vi "Initialize Instrument Engine.vi"(8 "error in (no error)":errorcluster, 9 "Name":string, 11 "Process":refnum<class "Process.lvclass">) -> (0 "error out":errorcluster, 2 "notification":bool, 3 "State Variables":T1)   [LabVIEW 2015, in "Instrument Addon Engine.lvlib"]
uses:
  Instrument Addon Engine.lvlib
  Types/Engine State Variables.ctl
  <vilib>/NI/NIVS Inline Async API/_VS Inline Async API/Process/Process.lvclass
  <vilib>/NI/NIVS Addon Network Comm/Engine/VeriStand Comm.lvclass
  <vilib>/NI/NIVS Inline Async API/_Data Access Engine/Access Type Classes/Write/Write.lvclass
  <vilib>/NI/NIVS Inline Async API/_Data Access Engine/Access Type Classes/Read/Read.lvclass
  <vilib>/NI/NIVS Inline Async API/_Data Access Engine/Access Type Classes/ReadWrite/ReadWrite.lvclass
  <vilib>/NI/NIVS Addon Network Comm/Engine/VeriStand Comm.lvclass/VeriStand Comm.ctl
  <vilib>/NI/NIVS Inline Async API/_VS Inline Async API/Process/Process.lvclass/Process.ctl
  <vilib>/NI/NIVS Inline Async API/_VS Inline Async API/Process/Data Member Access/Read Data Access.vi
  <vilib>/NI/NIVS Inline Async API/_VS Inline Async API/Error Handling Process/SubVIs/Error.ConvertArray.vi
  <vilib>/NI/NIVS Inline Async API/_Data Access Engine/Data Access Engine/Methods/Read.Lookup.vi
  <vilib>/NI/NIVS Inline Async API/_Data Access Engine/Data Access Engine/Methods/Write.Lookup.vi
  <vilib>/NI/NIVS Inline Async API/_Data Access Engine/Data Access Engine/Methods/ReadWrite.Lookup.vi
  <vilib>/NI/STM/Connection Manager/TCP/Advanced/TCP Initialize Connection Manager (By Reference).vi
  <vilib>/NI/AMC/Create Message Queue.vi
  Shared/Constants.vi
  <vilib>/NI/NIVS Inline Async API/_Data Access Engine/Data Access Engine/Data Access Engine.lvclass
  <vilib>/NI Veristand/Custom Device Tools/Custom Device Utility Library/Custom Device Utility Library.lvlib
  Shared/Instrument Addon Shared.lvlib
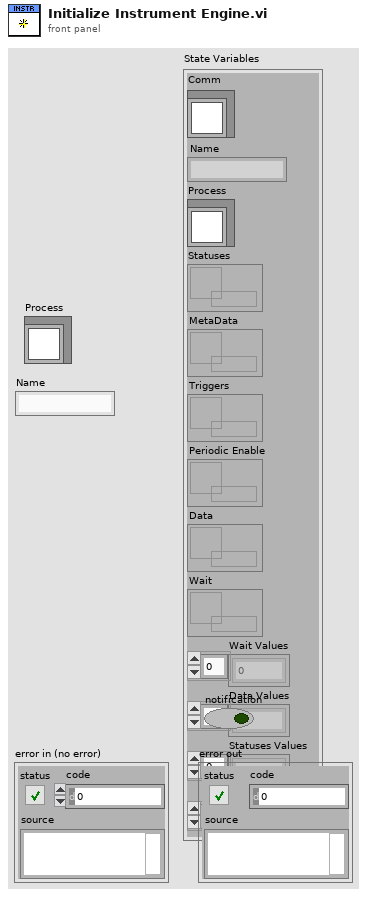
[diagram p1: front panel]
types:
  T1 = typedef "Instrument Addon Engine.lvlib/Engine State Variables.ctl" = cluster{"Comm":refnum<class "VeriStand Comm.lvclass">, "Name":string, "Process":refnum<class "Process.lvclass">, "Statuses":refnum<data-value>, "MetaData":refnum<data-value>, "Triggers":refnum<data-value>, "Periodic Enable":refnum<data-value>, "Data":refnum<data-value>, "Wait":refnum<data-value>, "Wait Values":dbl[], "Data Values":dbl[], "Statuses Values":dbl[], "MetaData Values":dbl[]}
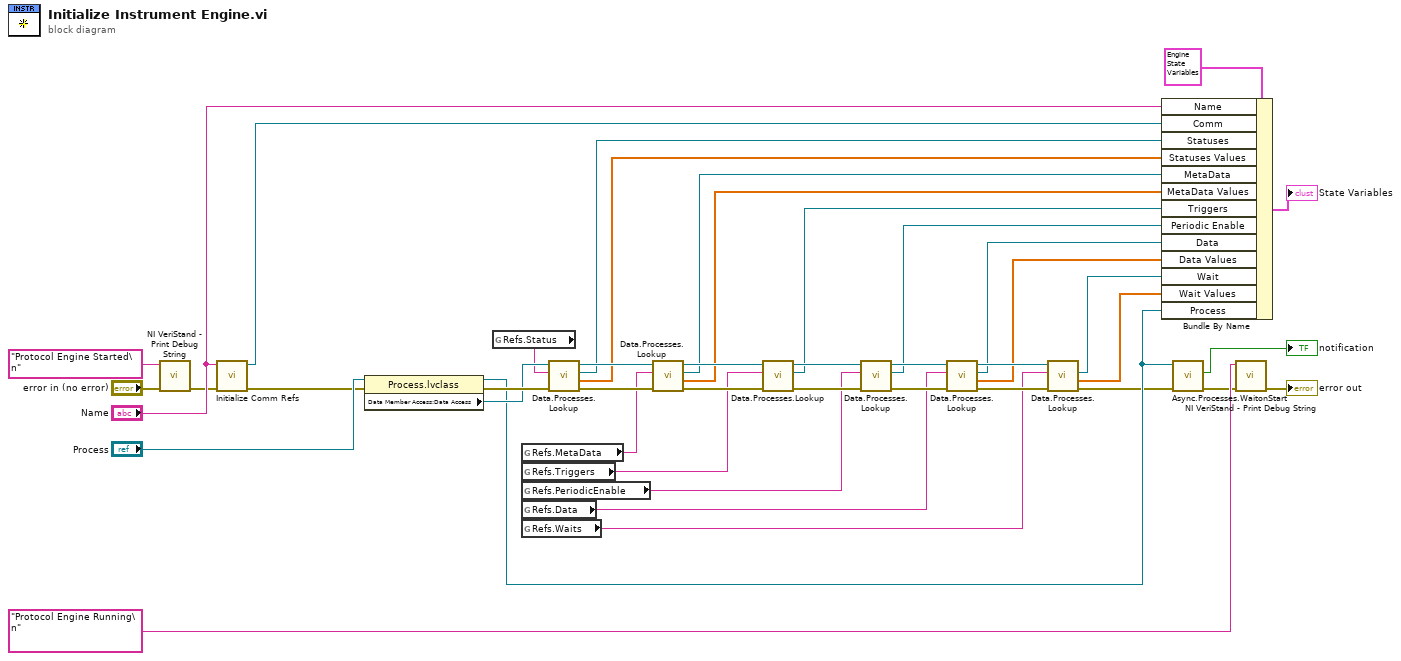
[diagram p0: block diagram]
diagram:
  n1 = call <vilib>:"NI VeriStand - Print Debug String.vi"("error in (no error)"="error in (no error)", "Message"="Protocol Engine Started\n" ("Debug String")) -> ("error out"=w33:errorcluster)  [unwired: 9 in]
  n2 = call <vilib>:"Initialize Comm Refs.vi"("error in (no error)"=w33, "Name"="Name") -> ("error out"=w2:errorcluster, "Comm.lvclass"=w41:refnum<class "VeriStand Comm.lvclass">)  [unwired: 8 in]
  n3 = property class="Process.lvclass"(reference="Process", error in=w2) -> (reference out=w24:refnum<class "Process.lvclass">, error out=w32:errorcluster, "Data Member Access:Data Access"=w31:refnum<class "Data Access Engine.lvclass">)
  n4 = global read "Constants.vi" "Refs.Status"() -> (w13:string)
  n5 = global read "Constants.vi" "Refs.MetaData"() -> (w12:string)
  n6 = global read "Constants.vi" "Refs.Triggers"() -> (w10:string)
  n7 = global read "Constants.vi" "Refs.PeriodicEnable"() -> (w9:string)
  n8 = global read "Constants.vi" "Refs.Data"() -> (w8:string)
  n9 = global read "Constants.vi" "Refs.Waits"() -> (w7:string)
  n10 = call-poly <vilib>:"Data.Processes.Lookup.vi"("error in (no error)"=w32, "Name"=w13, "Data Access API in"=w31) -> ("error out"=w14:errorcluster, "Initial Values"=w4:dbl[], "Ref"=w1:refnum<data-value>, "Data Access API out"=w30:refnum<class "Data Access Engine.lvclass">)  [unwired: 5 in]
  n11 = call-poly <vilib>:"Data.Processes.Lookup.vi"("error in (no error)"=w14, "Name"=w12, "Data Access API in"=w30) -> ("error out"=w11:errorcluster, "Initial Values"=w5:dbl[], "Ref"=w15:refnum<data-value>, "Data Access API out"=w29:refnum<class "Data Access Engine.lvclass">)  [unwired: 5 in]
  n12 = call-poly <vilib>:"Data.Processes.Lookup.vi"("error in (no error)"=w11, "Name"=w10, "Data Access API in"=w29) -> ("error out"=w17:errorcluster, "Ref"=w16:refnum<data-value>, "Data Access API out"=w28:refnum<class "Data Access Engine.lvclass">)  [unwired: 5 in, 1 out]
  n13 = call-poly <vilib>:"Data.Processes.Lookup.vi"("error in (no error)"=w17, "Name"=w9, "Data Access API in"=w28) -> ("error out"=w18:errorcluster, "Ref"=w19:refnum<data-value>, "Data Access API out"=w27:refnum<class "Data Access Engine.lvclass">)  [unwired: 5 in, 1 out]
  n14 = call-poly <vilib>:"Data.Processes.Lookup.vi"("error in (no error)"=w18, "Name"=w8, "Data Access API in"=w27) -> ("error out"=w20:errorcluster, "Initial Values"=w3:dbl[], "Ref"=w21:refnum<data-value>, "Data Access API out"=w26:refnum<class "Data Access Engine.lvclass">)  [unwired: 5 in]
  n15 = call-poly <vilib>:"Data.Processes.Lookup.vi"("error in (no error)"=w20, "Name"=w7, "Data Access API in"=w26) -> ("error out"=w23:errorcluster, "Initial Values"=w6:dbl[], "Ref"=w22:refnum<data-value>)  [unwired: 5 in, 1 out]
  n16 = Bundle By Name(cluster=T1 {"Comm"=refnum, "Name"="", "Process"=refnum, "Statuses"=refnum, "MetaData"=refnum, "Triggers"=refnum, "Periodic Enable"=refnum, "Data"=refnum, "Wait"=refnum, "Wait Values"=[], "Data Values"=[], "Statuses Values"=[], "MetaData Values"=[]} ("State Variables"), "Name"="Name", "Comm"=w41, "Statuses"=w1, "Statuses Values"=w4, "MetaData"=w15, "MetaData Values"=w5, "Triggers"=w16, "Periodic Enable"=w19, "Data"=w21, "Data Values"=w3, "Wait"=w22, "Wait Values"=w6, "Process"=w24) -> (→"State Variables":T1)
  n17 = call <vilib>:"Async.Processes.WaitonStart.vi"("error in (no error)"=w23, "Process"=w24) -> ("error out"=w35:errorcluster, "Execute"=→"notification":bool)  [unwired: 7 in, 1 out]
  n18 = call <vilib>:"NI VeriStand - Print Debug String.vi"("error in (no error)"=w35, "Message"="Protocol Engine Running\n" ("Debug String")) -> ("error out"=→"error out":errorcluster)  [unwired: 9 in]
